vi "RSZVB Get Calibration Data Type.vi"(8 "error in (no error)":errorcluster {"code" format="%.0x"}, 9 "Calibration (1)":i32=1, 10 "Channel (1)":i32=1, 11 "VISA session":refnum<visa-resource-name>) -> (0 "error out":errorcluster {"code" format="%.0x"}, 2 "Calibration Type":i32, 3 "dup VISA session":refnum<visa-resource-name>)   [LabVIEW 2011]
doc: "This VI queries the calibration type.\n\nRemote-control command(s):\n[SENSe<Ch>:]CORRection:DATA:PARameter<Cal>? TYPE"
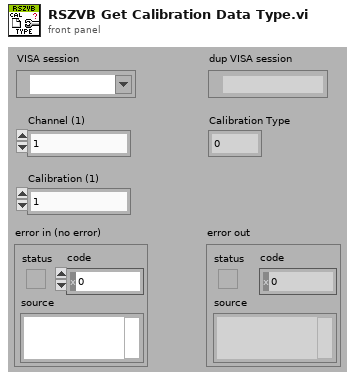
[diagram p1: front panel]
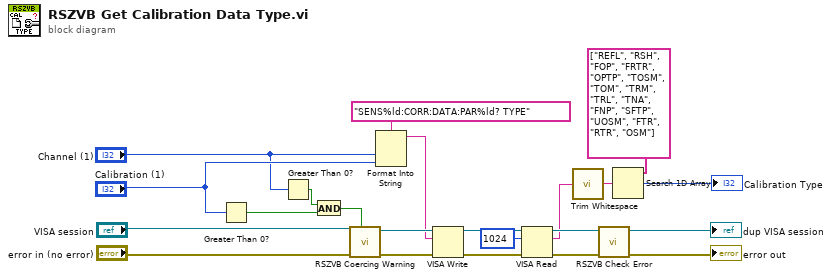
[diagram p0: block diagram]
diagram:
  n1 = Greater Than 0?(x="Calibration (1)") -> (x > 0?=w11:bool)
  n2 = Greater Than 0?(x="Channel (1)") -> (x > 0?=w12:bool)
  n3 = And(x=w12, y=w11) -> (x .and. y?=w13:bool)
  n4 = call "RSZVB Coercing Warning.vi"("In Range?"=w13, "error in (no error)"="error in (no error)", "VISA session"="VISA session") -> ("error out"=w16:errorcluster, "dup VISA session"=w17:refnum<visa-resource-name>)  [unwired: 7 in]
  n5 = Format Into String(format string="SENS%ld:CORR:DATA:PAR%ld? TYPE", "Channel (1)", "Calibration (1)") -> (resulting string=w14:string)  [unwired: 2 in, 1 out]
  n6 = VISA Write(VISA resource name=w17, write buffer=w14, error in (no error)=w16) -> (VISA resource name out=w21:refnum<visa-resource-name>, error out=w22:errorcluster)  [unwired: 1 out]
  n7 = VISA Read(VISA resource name=w21, byte count=u32 1024, error in (no error)=w22) -> (VISA resource name out=w18:refnum<visa-resource-name>, read buffer=w8:string, error out=w19:errorcluster)  [unwired: 1 out]
  n8 = call <vilib>:"Trim Whitespace.vi"("string"=w8) -> ("trimmed string"=w10:string)  [unwired: 1 in]
  n9 = call "RSZVB Check Error.vi"("error in (no error)"=w19, "VISA session"=w18) -> ("error out"=→"error out":errorcluster, "dup VISA session"=→"dup VISA session":refnum<visa-resource-name>)  [unwired: 8 in]
  n10 = Search 1D Array(1D array=string[] ["REFL", "RSH", "FOP", "FRTR", "OPTP", "TOSM", "TOM", "TRM", "TRL", "TNA", "FNP", "SFTP", "UOSM", "FTR", "RTR", "OSM"] ("array 2"), element=w10) -> (index of element=→"Calibration Type":i32)  [unwired: 1 in]
